vi "Configure Radio Standard.vi"(0 "VISA resource name":refnum<visa-resource-name>, 1 "Signal Bandwidth (3.0 MHz)":dbl=3000000.0 format="%#.6g", 2 "Band Class (0: BC0)":u16(ring) items=["BC0", "BC1"], 3 "Device BTS/MS (0: Base Transmitter Station)":u16(ring) items=["Base Transmitter Station", "Repeat"], 5 "Standard (0: None)":u16(ring) items=["None", "IS-95A", "J-STD-008", "IS-95C", "GSM/EDGE", "3GPP W-CDMA", "CDMA2000 MC-1X", "CDMA2000 DS", "CDMA2000 MC-3X", "NADC", "PDC", "Bluetooth", "TETRA", "802.11a", "802.11b", "802.11g", "Hiper LAN/2", "DVB-T", "G/PAL/NICAM", "I/PAL/NICAM", "FCC Part 15 Subpart F", "S-DMB", "UWB Indoor"], 7 "Enable All Measurements (Disable)":bool, 9 "Enable Retain Params  (Disable)":bool, 11 "error in (no error)":errorcluster, 12 "Packet Type (0: DH1)":u16(ring) items=["DH1", "DH3", "DH5"]) -> (4 "VISA resource name out":refnum<visa-resource-name>, 15 "error out":errorcluster)   [LabVIEW 2014, in "Agilent ESA PSA Series.lvlib"]
doc: "Configures the available radio standard."
uses:
  Agilent ESA PSA Series.lvlib
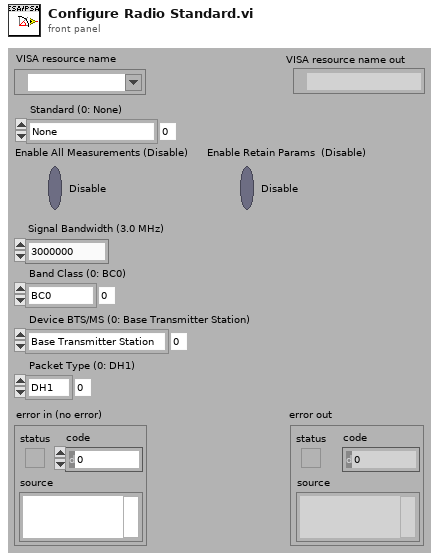
[diagram p1: front panel]
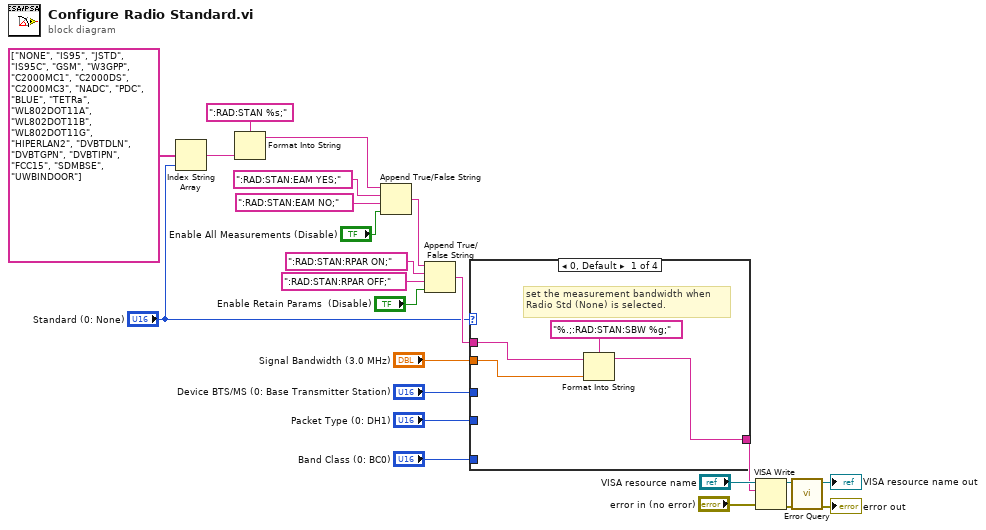
[diagram p0: block diagram]
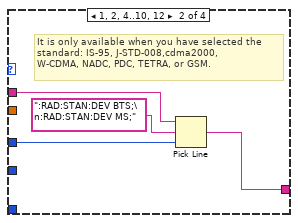
[diagram p2: hidden frame]
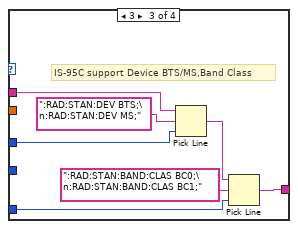
[diagram p3: hidden frame]
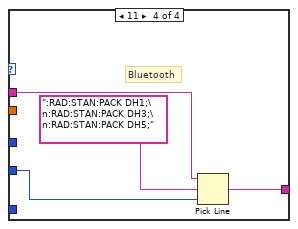
[diagram p4: hidden frame]
diagram:
  n1 = Index String Array(1:"Standard (0: None)", 2:string[] ["NONE", "IS95", "JSTD", "IS95C", "GSM", "W3GPP", "C2000MC1", "C2000DS", "C2000MC3", "NADC", "PDC", "BLUE", "TETRa", "WL802DOT11A", "WL802DOT11B", "WL802DOT11G", "HIPERLAN2", "DVBTDLN", "DVBTGPN", "DVBTIPN", "FCC15", "SDMBSE", "UWBINDOOR"]) -> (0:w23:string)  [unwired: 1 in]
  n2 = Format Into String(format string=":RAD:STAN %s;", w23) -> (resulting string=w18:string)  [unwired: 2 in, 1 out]
  n3 = Append True/False String(1:"Enable All Measurements (Disable)", 2:":RAD:STAN:EAM NO;" ("true string"), 3:":RAD:STAN:EAM YES;" ("true string"), 4:w18) -> (0:w17:string)
  n4 = Append True/False String(1:"Enable Retain Params  (Disable)", 2:":RAD:STAN:RPAR OFF;" ("true string"), 3:":RAD:STAN:RPAR ON;" ("true string"), 4:w17) -> (0:w13:string)
  n5 = case shown="0, Default" "Standard (0: None)" {
    tunnel: w13 -> [w28 w30 w37 w41]
    tunnel: "Signal Bandwidth (3.0 MHz)" -> [w26 _ _ _]
    tunnel: [w25 w29 w33 w42] -> w1
    tunnel: "Device BTS/MS (0: Base Transmitter Station)" -> [_ w31 w38 _]
    tunnel: "Packet Type (0: DH1)" -> [_ _ _ w40]
    tunnel: "Band Class (0: BC0)" -> [_ _ w34 _]
    frame 0, Default {
      # "set the measurement bandwidth when\nRadio Std (None) is selected."
      n6 = Format Into String(format string="%.;:RAD:STAN:SBW %g;", initial string=w28, w26) -> (resulting string=w25:string)  [unwired: 1 in, 1 out]
    }
    frame 1, 2, 4..10, 12 {
      # "It is only available when you have selected the \nstandard: IS-95, J-STD-008,cdma2000, \nW-CDMA, NADC, PDC, TETRA, or GSM."
      n7 = Pick Line(string ("")=w30, multi-line string=":RAD:STAN:DEV BTS;\n:RAD:STAN:DEV MS;", line index=w31) -> (output string=w29:string)
    }
    frame 3 {
      # "IS-95C support Device BTS/MS,Band Class"
      n8 = Pick Line(string ("")=w37, multi-line string=":RAD:STAN:DEV BTS;\n:RAD:STAN:DEV MS;", line index=w38) -> (output string=w35:string)
      n9 = Pick Line(string ("")=w35, multi-line string=":RAD:STAN:BAND:CLAS BC0;\n:RAD:STAN:BAND:CLAS BC1;", line index=w34) -> (output string=w33:string)
    }
    frame 11 {
      # "Bluetooth"
      n10 = Pick Line(string ("")=w41, multi-line string=":RAD:STAN:PACK DH1;\n:RAD:STAN:PACK DH3;\n:RAD:STAN:PACK DH5;", line index=w40) -> (output string=w42:string)
    }
  }
  n11 = VISA Write(VISA resource name="VISA resource name", write buffer=w1, error in (no error)="error in (no error)") -> (VISA resource name out=w10:refnum<visa-resource-name>, error out=w11:errorcluster)  [unwired: 1 out]
  n12 = call "Error Query.vi"("error in (no error)"=w11, "VISA resource name"=w10) -> ("error out"=→"error out":errorcluster, "VISA resource name out"=→"VISA resource name out":refnum<visa-resource-name>)  [unwired: 6 in, 2 out]
